vi "Main Database.vi"(8 "error in (no error)":errorcluster, 11 "Module_Refs":T1={"ModuleName"=enum."Controller", "Queue"=refnum, "user event"=refnum, "VI Refnum"=refnum, "ShowFP"=FALSE, "StatesTracking Enabled"=FALSE}) -> (0 "error out":errorcluster)   [LabVIEW 2019, in "Configuration Database.lvlib"]
doc: "Main Module Template of the architecture. Use this as a template to integrate new independent processes into your application."
uses:
  Configuration Database.lvlib
  Architecture/Typedefs/Enum_Module_Name.ctl
  Architecture/Architecture.lvlib
  Architecture/Typedefs/Message.ctl
  Architecture/Typedefs/Module References.ctl
  Typedefs/State Machine Data.ctl
  Architecture/Typedefs/Application Configuration.ctl
  Typedefs/Config.ctl
  Architecture/Modules/Module Template/SubVIs/Module Template Configuraton Extractor API.vi
  Architecture/Modules/Module Template/Typedefs/Config.ctl
  Architecture/Modules/Module Template/Module Template.lvlib
  Typedefs/Account.ctl
panel:
  in  "Stop App":bool
  out "Message":string
  in  "Stop Module":bool
  # "#Architecture\n\nPlace inside this box all visible data."
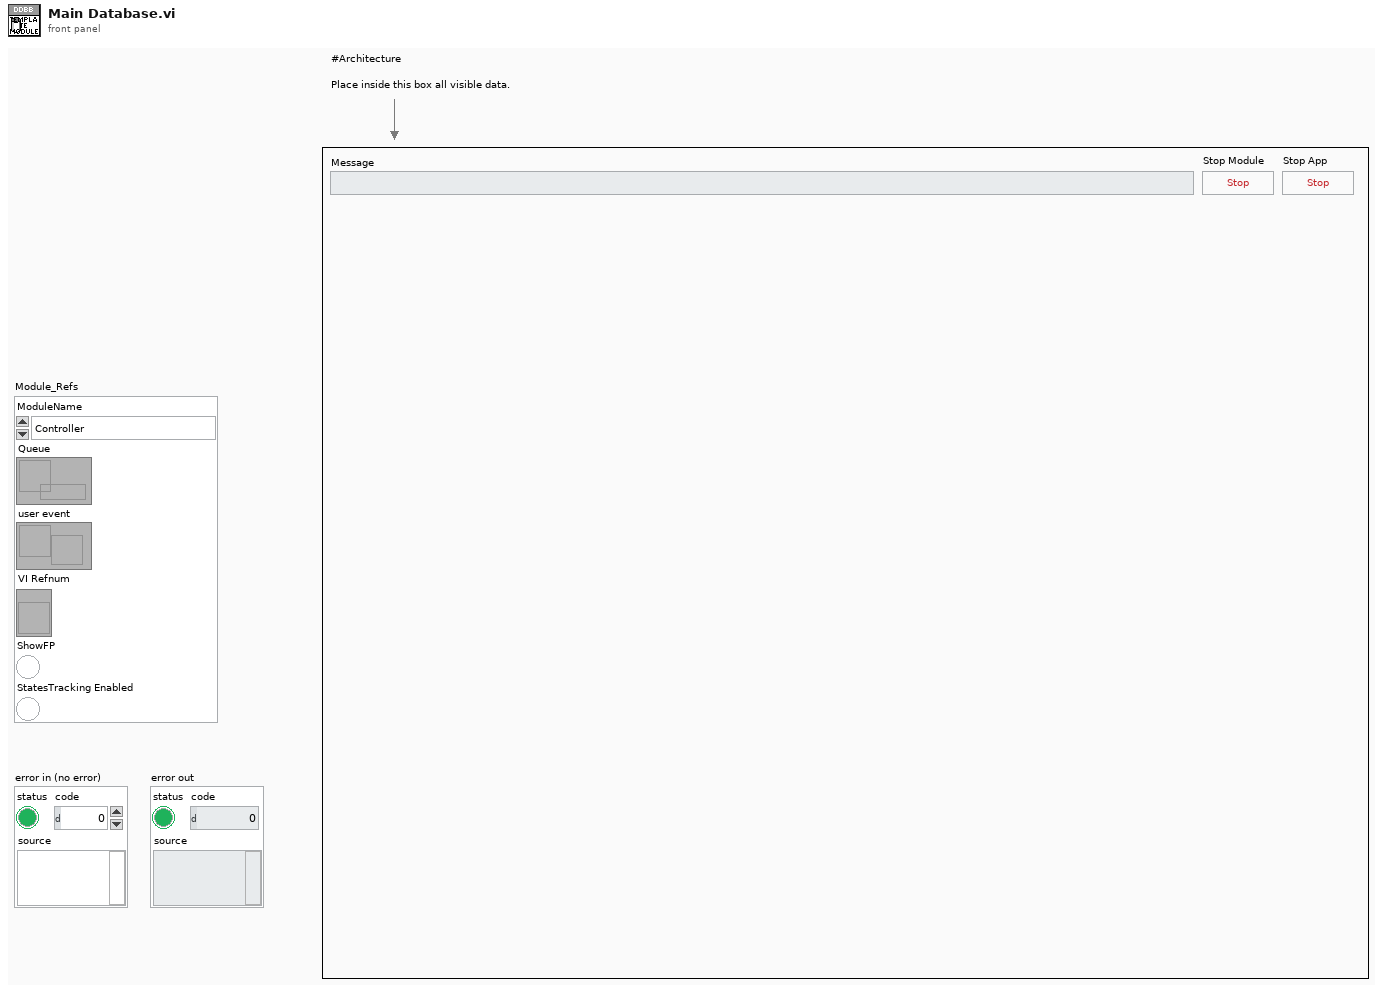
[diagram p1: front panel]
types:
  T1 = typedef "Architecture.lvlib/Module References.ctl" = cluster{"ModuleName":T2, "Queue":refnum<queue>, "user event":refnum<user-event>, "VI Refnum":refnum<vi>, "ShowFP":bool, "StatesTracking Enabled":bool}
  T2 = typedef "Architecture.lvlib/Enum_Module_Name.ctl" = enum16{"Configuration", "Error_Handler", "Log", "Database", "Controller", "User Console", "Display Console", "Sensor Interface"}
  T3 = typedef "Configuration Database.lvlib/State Machine Data.ctl" = cluster{"Module_Refs":T1, "Response Data":variant, "Module Template Config":T4, "Accounts":T5[]}
  T4 = typedef "Configuration Database.lvlib/Config.ctl" = cluster{"Module Enabled":bool}
  T5 = typedef "Configuration Database.lvlib/Account.ctl" = cluster{"Number":i32, "First Name":string, "Last Name":string, "Balance":dbl}
  T6 = enum32{"Invalid", "Standard", "Closed", "Hidden", "Minimized", "Maximized"}
  T7 = typedef "Architecture.lvlib/Module Template.lvlib/Config.ctl" = cluster{"Module Enabled":bool}
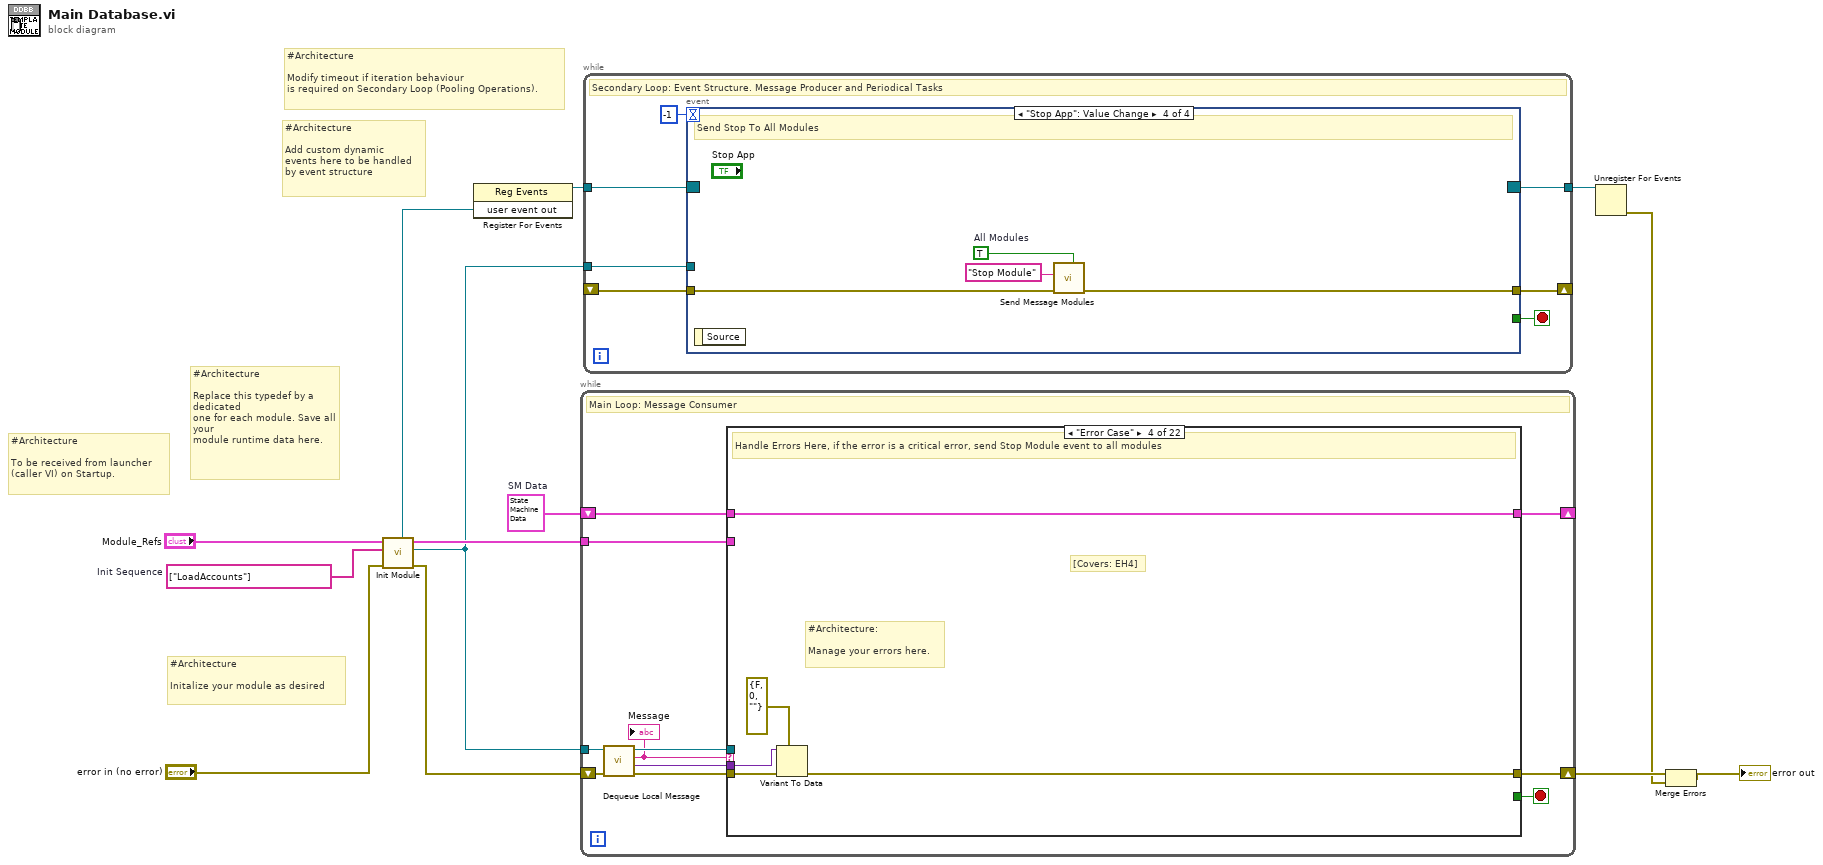
[diagram p0: block diagram]
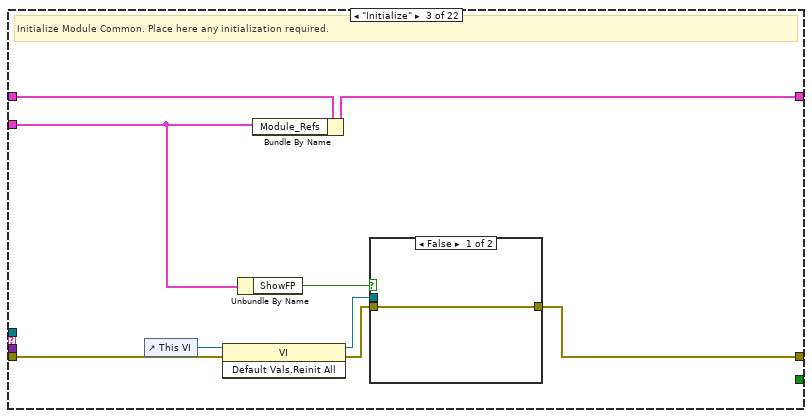
[diagram p4: hidden frame]
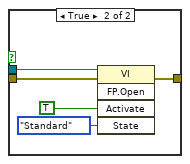
[diagram p5: hidden frame]
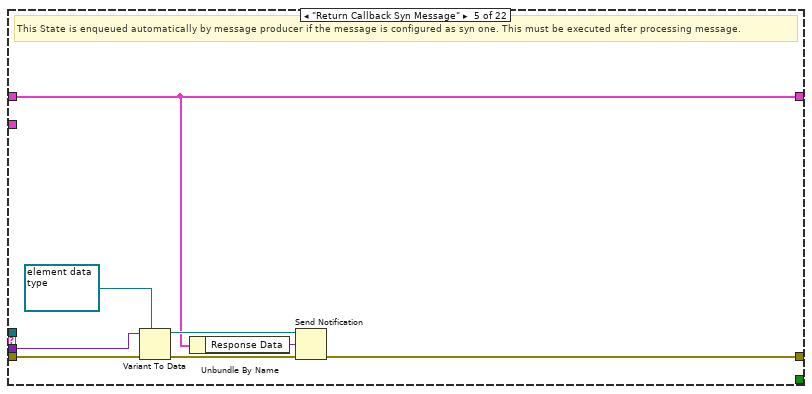
[diagram p6: hidden frame]
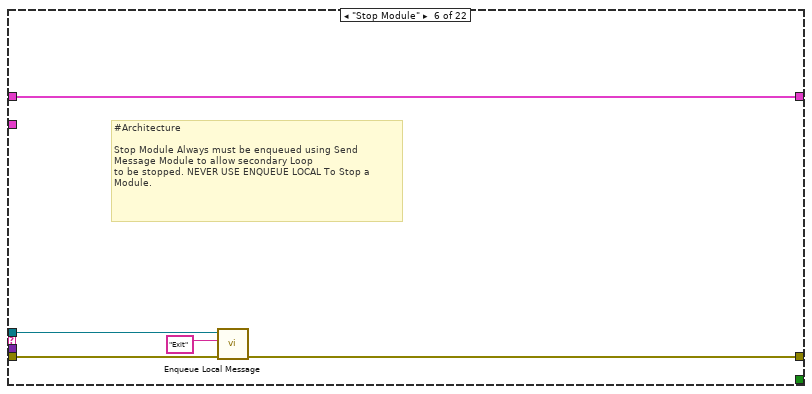
[diagram p7: hidden frame]
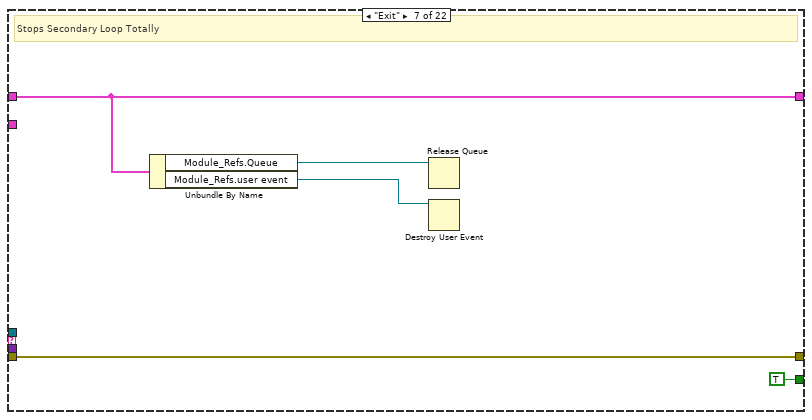
[diagram p8: hidden frame]
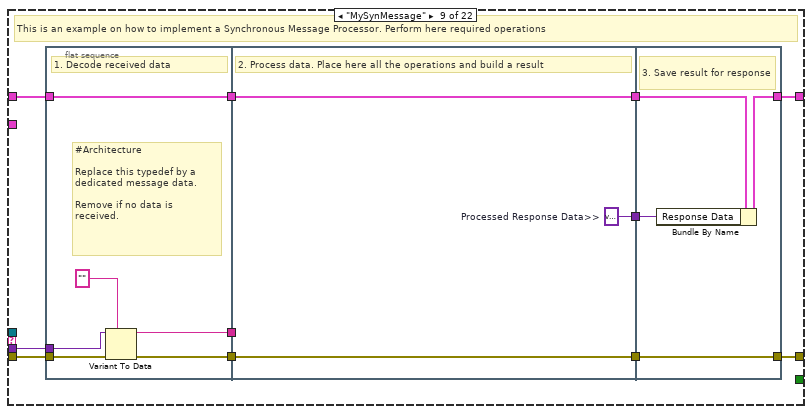
[diagram p10: hidden frame]
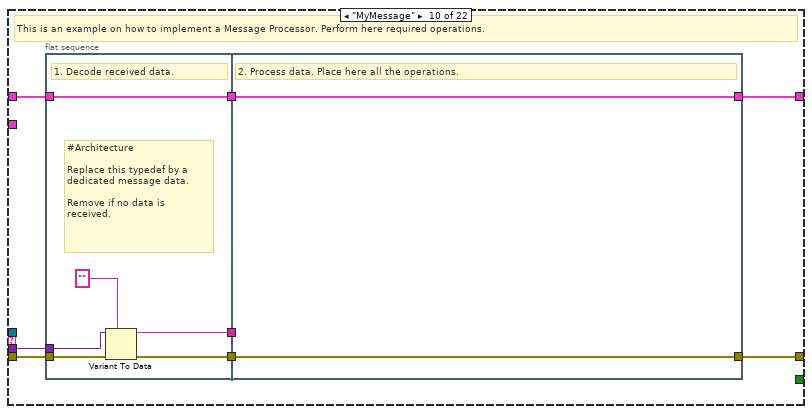
[diagram p11: hidden frame]
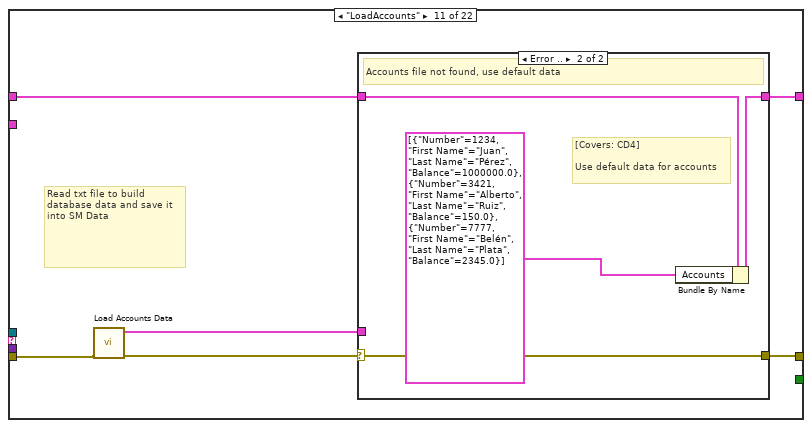
[diagram p12: hidden frame]
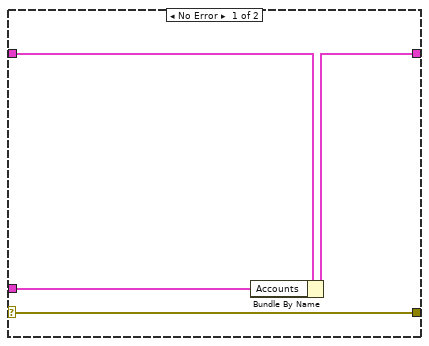
[diagram p13: hidden frame]
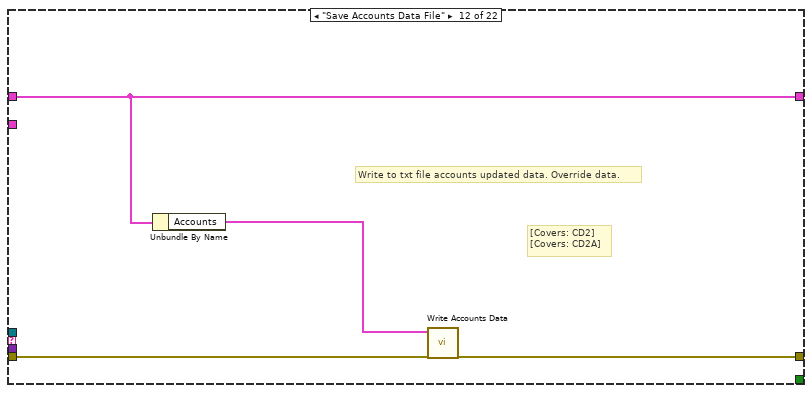
[diagram p14: hidden frame]
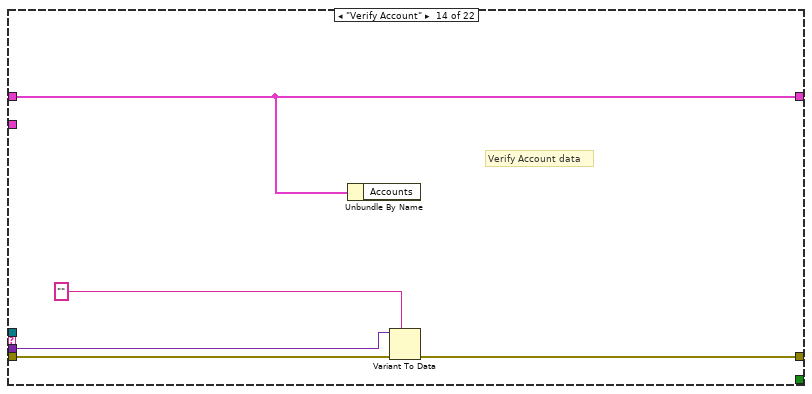
[diagram p16: hidden frame]
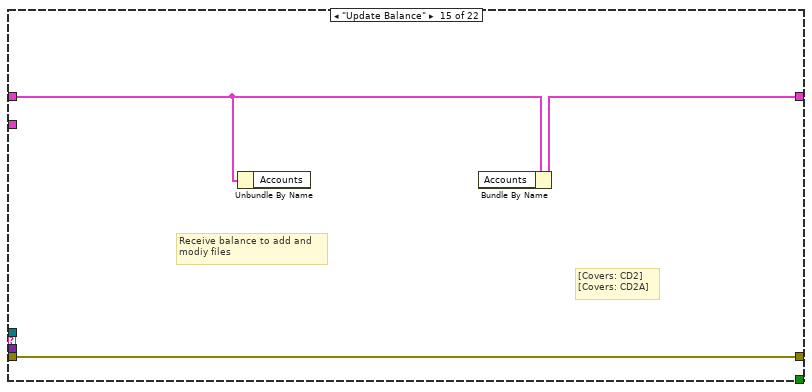
[diagram p17: hidden frame]
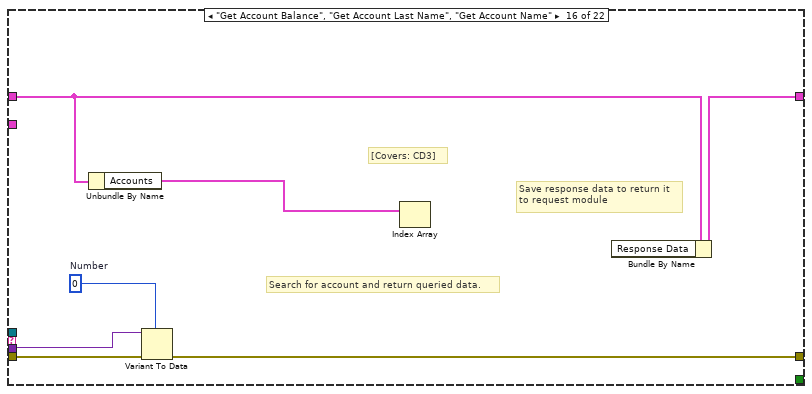
[diagram p18: hidden frame]
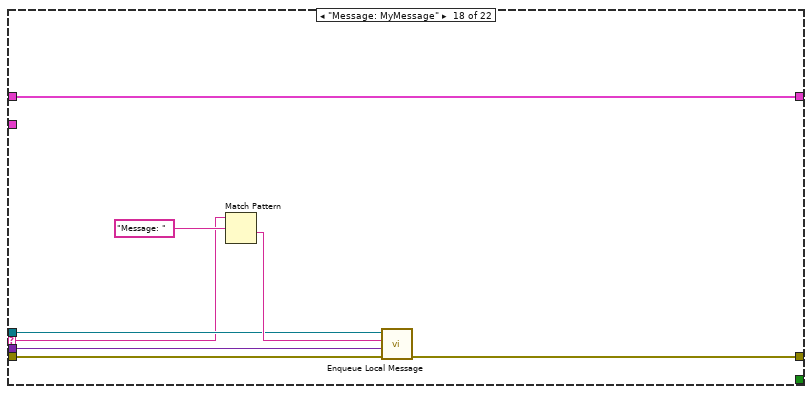
[diagram p20: hidden frame]
diagram:
  w10 = string[] ["LoadAccounts"]  # Init Sequence
  w13 = T3 {"Module_Refs"={"ModuleName"=enum."Controller", "Queue"=refnum, "user event"=refnum, "VI Refnum"=refnum, "ShowFP"=FALSE, "StatesTracking Enabled"=FALSE}, "Response Data"=variant, "Module Template Config"={"Module Enabled"=FALSE}, "Accounts"=[]}  # SM Data
  # "#Architecture\n\nModify timeout if iteration behaviour \nis required on Secondary Loop (Pooling Operations)."
  # "#Architecture\n\nAdd custom dynamic \nevents here to be handled \nby event structure"
  # "#Architecture\n\nInitalize your module as desired"
  # "#Architecture\n\nTo be received from launcher \n(caller VI) on Startup."
  # "#Architecture\n\nReplace this typedef by a dedicated \none for each module. Save all your \nmodule runtime data here."
  n1 = call "Init Module.vi"("error in (no error)"="error in (no error)", "Init Sequence"=w10, "Module Refs"="Module_Refs") -> ("error out"=w12:errorcluster, "queue out"=w1:refnum<queue>, "Module Refs Out"=w3:T1, "user event out"=w2:refnum<user-event>)  [unwired: 5 in]
  n2 = register-events(w2) -> (reference out=w9:refnum<event-registration>)  [unwired: 2 in, 1 out]
  n3 = while {
    shift-right: [w23] -> _
    shift-left: w13 -> [w24]
    shift-right: [w22] -> w7
    shift-left: w12 -> [w20]
    tunnel: w1 -> [w21]
    tunnel: w3 -> [w14]
    stop <- w15 stop-if-true
    # "Main Loop: Message Consumer"
    n4 = call "Dequeue Local Message.vi"("error in"=w20, "Msg queue in"=w21) -> ("error out"=w19:errorcluster, "Data"=w16:variant, "Message"=w17:string, "queue out"=w18:refnum<queue>)  [unwired: 6 in]
    "Message" <- w17
    n5 = case shown="\"Error Case\"" w17 {
      selector: w17 -> [_ _ _ _ _ _ _ _ _ _ _ _ _ _ _ _ _ w145 _ _ _ w177]
      tunnel: w24 -> [w26 w28 w37 w48 w50 w61 w64 w68 w79 w100 w114 w124 w127 w128 w134 w141 w144 w152 w157 w166 w168 w182]
      tunnel: [w26 w28 w35 w48 w50 w61 w64 w68 w78 w93 w112 w124 w127 w128 w133 w136 w144 w152 w157 w159 w168 w182] -> w23
      tunnel: w19 -> [w25 w27 w36 w47 w56 w60 w66 w67 w72 w96 w113 w125 w126 w132 w135 w142 w143 w149 w156 w165 w167 w181]
      tunnel: [w25 w27 w31 w46 w55 w59 w66 w67 w77 w99 w109 w125 w126 w131 w135 w140 w143 w146 w155 w160 w167 w171] -> w22
      tunnel: w18 -> [_ _ _ _ _ w58 _ _ _ _ _ _ _ _ _ _ _ w147 w154 _ _ w178]
      tunnel: w16 -> [_ _ _ w45 w53 _ _ _ w71 w95 _ _ _ w129 _ w138 _ w148 _ w164 _ w179]
      tunnel: [_ _ _ _ _ _ TRUE _ _ _ _ _ _ _ _ _ _ _ _ _ _ _] -> w15
      tunnel: w14 -> [_ _ w34 _ _ _ _ _ _ _ _ _ _ _ _ _ _ _ _ _ _ _]
      frame "--------State Machine Arquitechture Operations--------" {
      }
      frame "Idle", Default {
        # "Use this state to make iterations if required."
      }
      frame "Initialize" {
        # "Initialize Module Common. Place here any initialization required."
        n6 = control-ref of="This VI"() -> (w29:refnum<vi>)
        n7 = invoke class="VI" method="Default Vals.Reinit All"(reference=w29, error in=w36) -> (reference out=w32:refnum<vi>, error out=w33:errorcluster)  [unwired: 1 in, 1 out]
        n8 = Unbundle By Name(w34) -> ("ShowFP"=w30:bool)
        n9 = Bundle By Name(cluster=w37, "Module_Refs"=w34) -> (w35:T3)
        n10 = case shown="False" w30 {
          tunnel: w33 -> [w38 w43]
          tunnel: [w38 w42] -> w31
          tunnel: w32 -> [_ w41]
          frame False {
          }
          frame True {
            n11 = invoke class="VI" method="FP.Open"(reference=w41, error in=w43, "Activate"=TRUE ("Activate?"), "State"=T6."Standard") -> (error out=w42:errorcluster)  [unwired: 1 in, 4 out]
          }
        }
      }
      frame "Error Case" {
        # "[Covers: EH4]"
        # "#Architecture: \n\nManage your errors here."
        # "Handle Errors Here, if the error is a critical error, send Stop Module event to all modules"
        n12 = Variant To Data(error in=w47, type=errorcluster {"status"=FALSE, "code"=0, "source"=""} ("error constant"), Variant=w45) -> (error out=w46:errorcluster)  [unwired: 1 out]
      }
      frame "Return Callback Syn Message" {
        # "This State is enqueued automatically by message producer if the message is configured as syn one. This must be executed after processing message."
        n13 = Variant To Data(error in=w56, type=refnum<notifier> refnum ("notifier out"), Variant=w53) -> (data=w51:refnum<notifier>, error out=w54:errorcluster)
        n14 = Unbundle By Name(w50) -> ("Response Data"=w49:variant)
        n15 = Send Notification(notification=w49, notifier=w51, error in (no error)=w54) -> (error out=w55:errorcluster)  [unwired: 1 out]
      }
      frame "Stop Module" {
        # "#Architecture\n\nStop Module Always must be enqueued using Send Message Module to allow secondary Loop\nto be stopped. NEVER USE ENQUEUE LOCAL To Stop a Module."
        n16 = call "Enqueue Local Message.vi"("error in"=w60, "Message"="Exit", "Msg queue in"=w58) -> ("error out"=w59:errorcluster)  [unwired: 7 in, 1 out]
      }
      frame "Exit" {
        # "Stops Secondary Loop Totally"
        n17 = Unbundle By Name(w64) -> ("Module_Refs.Queue"=w63:refnum<queue>, "Module_Refs.user event"=w62:refnum<user-event>)
        n18 = Release Queue(queue=w63) -> ()  [unwired: 2 in, 3 out]
        n19 = Destroy User Event(user event=w62) -> ()  [unwired: 1 in, 1 out]
      }
      frame "--------------State Machine Custom States-------------" {
      }
      frame "MySynMessage" {
        # "This is an example on how to implement a Synchronous Message Processor. Perform here required operations"
        n20 = flat-sequence {
          tunnel: w72 -> [w83]
          tunnel: w79 -> [w85]
          tunnel: [w85] -> w76
          tunnel: [w81] -> w75
          tunnel: w71 -> [w82]
          tunnel: [w80] -> w70
          tunnel: w76 -> [w88]
          tunnel: w75 -> [w87]
          tunnel: [w88] -> w74
          tunnel: [w87] -> w73
          tunnel: w70 -> [_]
          tunnel: [w86] -> w69
          tunnel: [w91] -> w77
          tunnel: [w90] -> w78
          tunnel: w74 -> [w92]
          tunnel: w73 -> [w91]
          tunnel: w69 -> [w89]
          frame #0 {
            # "#Architecture\n\nReplace this typedef by a dedicated message data.\n\nRemove if no data is received."
            # "1. Decode received data"
            n21 = Variant To Data(error in=w83, type="", Variant=w82) -> (data=w80:string, error out=w81:errorcluster)
          }
          frame #1 {
            w86 = variant  # Processed Response Data>>
            # "2. Process data. Place here all the operations and build a result"
          }
          frame #2 {
            # "3. Save result for response"
            n22 = Bundle By Name(cluster=w92, "Response Data"=w89) -> (w90:T3)
          }
        }
      }
      frame "MyMessage" {
        # "This is an example on how to implement a Message Processor. Perform here required operations."
        n23 = flat-sequence {
          tunnel: w96 -> [w104]
          tunnel: w100 -> [w106]
          tunnel: [w106] -> w98
          tunnel: [w102] -> w97
          tunnel: w95 -> [w103]
          tunnel: [w101] -> w94
          tunnel: w98 -> [w107]
          tunnel: w97 -> [w108]
          tunnel: w94 -> [_]
          tunnel: [w108] -> w99
          tunnel: [w107] -> w93
          frame #0 {
            # "#Architecture\n\nReplace this typedef by a dedicated message data.\n\nRemove if no data is received."
            # "1. Decode received data."
            n24 = Variant To Data(error in=w104, type="", Variant=w103) -> (data=w101:string, error out=w102:errorcluster)
          }
          frame #1 {
            # "2. Process data. Place here all the operations."
          }
        }
      }
      frame "LoadAccounts" {
        # "Read txt file to build database data and save it into SM Data"
        n25 = call "Load Accounts Data.vi"("error in"=w113) -> ("error out"=w110:errorcluster, "Accounts"=w111:T5[])  [unwired: 9 in]
        n26 = case shown="Error .." w110 {
          selector: w110 -> [w115 w122]
          tunnel: w114 -> [w118 w121]
          tunnel: [w117 w120] -> w112
          tunnel: w111 -> [w116 _]
          tunnel: [w115 w122] -> w109
          frame No Error {
            n27 = Bundle By Name(cluster=w118, "Accounts"=w116) -> (w117:T3)
          }
          frame Error {
            # "[Covers: CD4] \n\nUse default data for accounts"
            # "Accounts file not found, use default data"
            n28 = Bundle By Name(cluster=w121, "Accounts"=T5[] [{"Number"=1234, "First Name"="Juan", "Last Name"="Pérez", "Balance"=1000000.0}, {"Number"=3421, "First Name"="Alberto", "Last Name"="Ruiz", "Balance"=150.0}, {"Number"=7777, "First Name"="Belén", "Last Name"="Plata", "Balance"=2345.0}]) -> (w120:T3)
          }
        }
      }
      frame "Save Accounts Data File" {
        # "[Covers: CD2] \n[Covers: CD2A]"
        # "Write to txt file accounts updated data. Override data."
        n29 = Unbundle By Name(w124) -> ("Accounts"=w123:T5[])
        n30 = call "Write Accounts Data.vi"("Accounts"=w123) -> ()  [unwired: 10 in, 1 out]
      }
      frame "Get Message" {
        # "[Covers: UM1A]\n\nBuild message from message id received from controller and send it \nback."
      }
      frame "Verify Account" {
        # "Verify Account data"
        n31 = Unbundle By Name(w128) -> ()  [unwired: 1 out]
        n32 = Variant To Data(error in=w132, type="", Variant=w129) -> (error out=w131:errorcluster)  [unwired: 1 out]
      }
      frame "Update Balance" {
        # "[Covers: CD2] \n[Covers: CD2A]"
        # "Receive balance to add and \nmodiy files"
        n33 = Unbundle By Name(w134) -> ()  [unwired: 1 out]
        n34 = Bundle By Name(cluster=w134) -> (w133:T3)  [unwired: 1 in]
      }
      frame "Get Account Balance", "Get Account Last Name", "Get Account Name" {
        w139 = 0  # Number
        # "[Covers: CD3]"
        # "Save response data to return it \nto request module"
        # "Search for account and return queried data."
        n35 = Unbundle By Name(w141) -> ("Accounts"=w137:T5[])
        n36 = Variant To Data(error in=w142, type=w139, Variant=w138) -> (error out=w140:errorcluster)  [unwired: 1 out]
        n37 = Index Array(array=w137) -> ()  [unwired: 1 in, 1 out]
        n38 = Bundle By Name(cluster=w141) -> (w136:T3)  [unwired: 1 in]
      }
      frame "--------------Dynamic Events Messages----------------" {
      }
      frame "Message: MyMessage" {
        n39 = Match Pattern(string=w145, regular expression="Message: ") -> (after substring=w150:string)  [unwired: 1 in, 3 out]
        n40 = call "Enqueue Local Message.vi"("error in"=w149, "Data"=w148, "Message"=w150, "Msg queue in"=w147) -> ("error out"=w146:errorcluster)  [unwired: 6 in, 1 out]
      }
      frame "Message: Stop Module" {
        n41 = call "Enqueue Local Message.vi"("error in"=w156, "Message"="Stop Module", "Msg queue in"=w154) -> ("error out"=w155:errorcluster)  [unwired: 7 in, 1 out]
      }
      frame "Message: Load Config" {
        # "Get dedicated data for this module from \ngeneral DVR configuration and save it into \nSM Data to use it on runtime."
        # "Message used to receive configuration from a configuration module. Decode dedicated typedef and save it into SM Data"
        n42 = Variant To Data(error in=w165, type=refnum<data-value> refnum ("data value reference"), Variant=w164) -> (data=w162:refnum<data-value>, error out=w161:errorcluster)
        n43 = call-poly "Read Configuration API.vi"("error constant"=w161, "General Config DVR In"=w162) -> ("error out"=w160:errorcluster, "Module Template Config"=w158:T7)  [unwired: 8 in]
        n44 = Bundle By Name(cluster=w166, "Module Template Config"=w158) -> (w159:T3)
      }
      frame "------------Synchronous Event Messages--------------" {
      }
      frame "SynMessage: Get Account Balance", "SynMessage: Get Account Last Name", "SynMessage: Get Account Name", "SynMessage: Get Message", "SynMessage: MySynMessage" {
        # "Use this case as a handler for Synchronous messages. This state queues a message for the desired"
        n45 = call "Extract Synchronous Data.vi"("error in 2"=w181, "Variant"=w179) -> ("error in"=w180:errorcluster, "Data Out"=w174:variant, "notifier out"=w169:refnum<notifier>)  [unwired: 7 in]
        n46 = Match Pattern(string=w177, regular expression="SynMessage: ") -> (after substring=w175:string)  [unwired: 1 in, 3 out]
        n47 = call "Enqueue Local Message.vi"("error in"=w180, "Data"=w174, "Message"=w175, "Msg queue in"=w178) -> ("error out"=w173:errorcluster, "queue out"=w172:refnum<queue>)  [unwired: 6 in]
        n48 = call "Enqueue Local Message.vi"("error in"=w173, "Data"=w169, "Message"="Return Callback Syn Message", "Msg queue in"=w172) -> ("error out"=w171:errorcluster)  [unwired: 6 in, 1 out]
      }
    }
  }
  n49 = while {
    tunnel: w9 -> [w189]
    tunnel: w1 -> [w186]
    tunnel: [w185] -> w8
    shift-right: [w183] -> _
    shift-left: _ -> [w184]
    stop <- w187 stop-if-true
    # "Secondary Loop: Event Structure. Message Producer and Periodical Tasks"
    n50 = event shown="[3] \"Stop App\": Value Change" {
      selector: w189 -> [_ _ _ _]
      dyn-events: [_ _ _ _] -> w185
      timeout: -1 -> [_ _ _ _]
      tunnel: [FALSE w198 TRUE _] -> w187
      tunnel: w186 -> [_ w203 w205 _]
      tunnel: w184 -> [w190 w202 w208 w210]
      tunnel: [w190 w201 w206 w209] -> w183
      event Timeout {
        n51 = event-data() -> ()  [unwired: 1 in, 1 out]
      }
      event User Event {
        # "Send message to local queue. \n(Message Consumer)"
        # "Processes an external event and enqueues a message to the local queue. It can be synchronous (with response) or NOT."
        n52 = event-data() -> ("syn"=w195:bool, "Message"=w197:string, "Data"=w200:variant)  [unwired: 1 in]
        n53 = Select(t="SynMessage: " ("string"), s=w195, f="Message: " ("string")) -> (s? t:f=w192:string)
        n54 = Concatenate Strings(w192, w197) -> (w199:string)
        n55 = call "Enqueue Local Message.vi"("error in"=w202, "Data"=w200, "Message"=w199, "Msg queue in"=w203) -> ("error out"=w201:errorcluster)  [unwired: 6 in, 1 out]
        n56 = Equal?(x=w197, y="Stop Module") -> (x = y?=w198:bool)
      }
      event "Stop Module": Value Change {
        n57 = event-data() -> ()  [unwired: 1 in, 1 out]
        n58 = call "Enqueue Local Message.vi"("error in"=w208, "Message"="Stop Module", "Msg queue in"=w205) -> ("error out"=w206:errorcluster)  [unwired: 7 in, 1 out]
      }
      event "Stop App": Value Change {
        w212 = TRUE  # All Modules
        # "Send Stop To All Modules"
        n59 = event-data() -> ()  [unwired: 1 in, 1 out]
        n60 = call "Send Message Modules.vi"("All Modules"=w212, "Error In"=w210, "Message"="Stop Module") -> ("error in (no error)"=w209:errorcluster)  [unwired: 8 in]
      }
    }
  }
  n61 = Unregister For Events(event registration refnum=w8) -> (error out=w6:errorcluster)  [unwired: 1 in]
  n62 = Merge Errors(w7, w6) -> (→"error out":errorcluster)
